vi "Uframe-Basler-MNR.vi"() -> ()   [LabVIEW 2010]
uses:
  <vilib>/userDefined/High Color/IMAQdx.ctl
  <vilib>/vision/driver/IMAQdx.llb/IMAQdx Buffer Number Mode.ctl
  <vilib>/Platform/TimedLoop/XDataNode/XDataNode.xnode
  <vilib>/Platform/TimedLoop/XDataNode/timing_clust.ctl
  <vilib>/Platform/TimedLoop/XDataNode/nitl_modes.ctl
  <vilib>/Platform/TimedLoop/XDataNode/wakeup.ctl
  <vilib>/Platform/TimedLoop/XDataNode/XDNodeRunTimeDep.lvlib
  <vilib>/vision/driver/NI_Vision_Acquisition_Software.lvlib
  Program Files/National Instruments/LabVIEW 2010/resource/objmgr/imaqdx.rc
panel:
  out "Load Cell Constant (N/V)":dbl=44.48
  in  "Load Cell":u16(ring)=1 items=["440 N", "1250 N"]
  in  "Pause @ Load":bool
  in  "Pause @ N":dbl
  out "Disp (mm)":dbl
  out "Load (N)":dbl
  out "Image #":i32
  in  "White Balance \nVR":dbl(slide)=1684.0 min=0.0 max=4095.0 step=1.0 scale=1.0..255.0 scale format="%#.0f"
  in  "White Balance\n UB":dbl(slide)=1684.0 min=0.0 max=4095.0 step=1.0 scale=1.0..255.0 scale format="%#.0f"
  in  "Illumination":u32(ring) items=["White Light", "Flourescent"]
  in  "Timed \nAcquisition":bool
  out "Data Point":i32
  in  "Shutter":dbl(slide)=20.0 min=0.0 max=4095.0 step=1.0 scale=4.095..4095.0 scale format="%#.0f"
  in  "Brightness":dbl(slide)=200.0 min=0.0 max=255.0 step=1.0 scale=0.0..255.0
  in  "Gain":dbl(slide)=702.0 min=350.0 max=1000.0 step=1.0 scale=350.0..1000.0
  in  "Video Mode Top":u32(ring)=47 items=["320x240 Color"=4, "640x480 Mono8"=9, "640x480 Mono16"=19, "640x480 Color"=14, "800x600 Mono8"=21, "800x600 Mono16"=27, "800x600 Color"=24, "1024x768 Mono8"=30, "1024x768 Mono16"=36, "1024x768 Color"=33, "1280x960 Mono8"=40, "1280x960 Mono16"=46, "1280x960 Color"=43, "1388x1038 Color"=47, "1388x1038 Mono"=48]
  in  "Session In Top View":T1="cam0"
  in  "Data \nAcquisition \nInterval (s)":dbl=1.0 min=0.1 max=60.0
  in  "Capture\nCurrent Image":bool
  out "Image":T2(plugin-control)
  in  "Max Load (N)":dbl=600.0 min=0.0 max=1200.0
  out "At Limit":bool
  in  "Rate Multiplier":dbl=1.0
  in  "Pause \nDisplacement":bool
  in  "Stop":bool
  in  "Invert \nDisplacement":bool
  in  "Zero \nDisplacement":bool=TRUE
  in  "Begin":bool
  out "Load vs Disp":cluster{dbl[], dbl[]}(graph)={[-724.1250113144533, -724.195323815552, -724.2656363166506, -724.3359488177492, -724.4062613188479, -724.4765738199465, -724.5468863210451, -724.6171988221438, -724.7461050741579, -724.9218863269045, -725.0976675796511, -725.2851675825808, -725.4492300851442], [-11.89350874713131, -11.896152101474941, -11.894229661847117, -11.89350874707076, -11.890865392620372, -11.895671491596438, -11.895911796524977, -11.899756675680168, -11.899035760801853, -11.90552399441818, -11.907927043887174, -11.905283689458143, -11.914655582386047]}
  out "Disp Vs Time":cluster{dbl[], dbl[]}(graph)={[-724.1250113144533, -724.195323815552, -724.2656363166506, -724.3359488177492, -724.4062613188479, -724.4765738199465, -724.5468863210451, -724.6171988221438, -724.7461050741579, -724.9218863269045, -725.0976675796511, -725.2851675825808, -725.4492300851442], [-11.89350874713131, -11.896152101474941, -11.894229661847117, -11.89350874707076, -11.890865392620372, -11.895671491596438, -11.895911796524977, -11.899756675680168, -11.899035760801853, -11.90552399441818, -11.907927043887174, -11.905283689458143, -11.914655582386047]}
  in  "File Name":string="Test"
  in  "File Path":path=path "C:/cygwin/home/Smarter Materials/Users 2015/Michael Rossol"
  in  "Sample Notes":string
  in  "Displacement \nRate (um/s)":dbl=3.0 min=3.0 max=50.0
  in  "Data Acquisition \nInterval (s)":dbl=1.0 min=0.1 max=10.0 step=0.01 format="%#_3g"
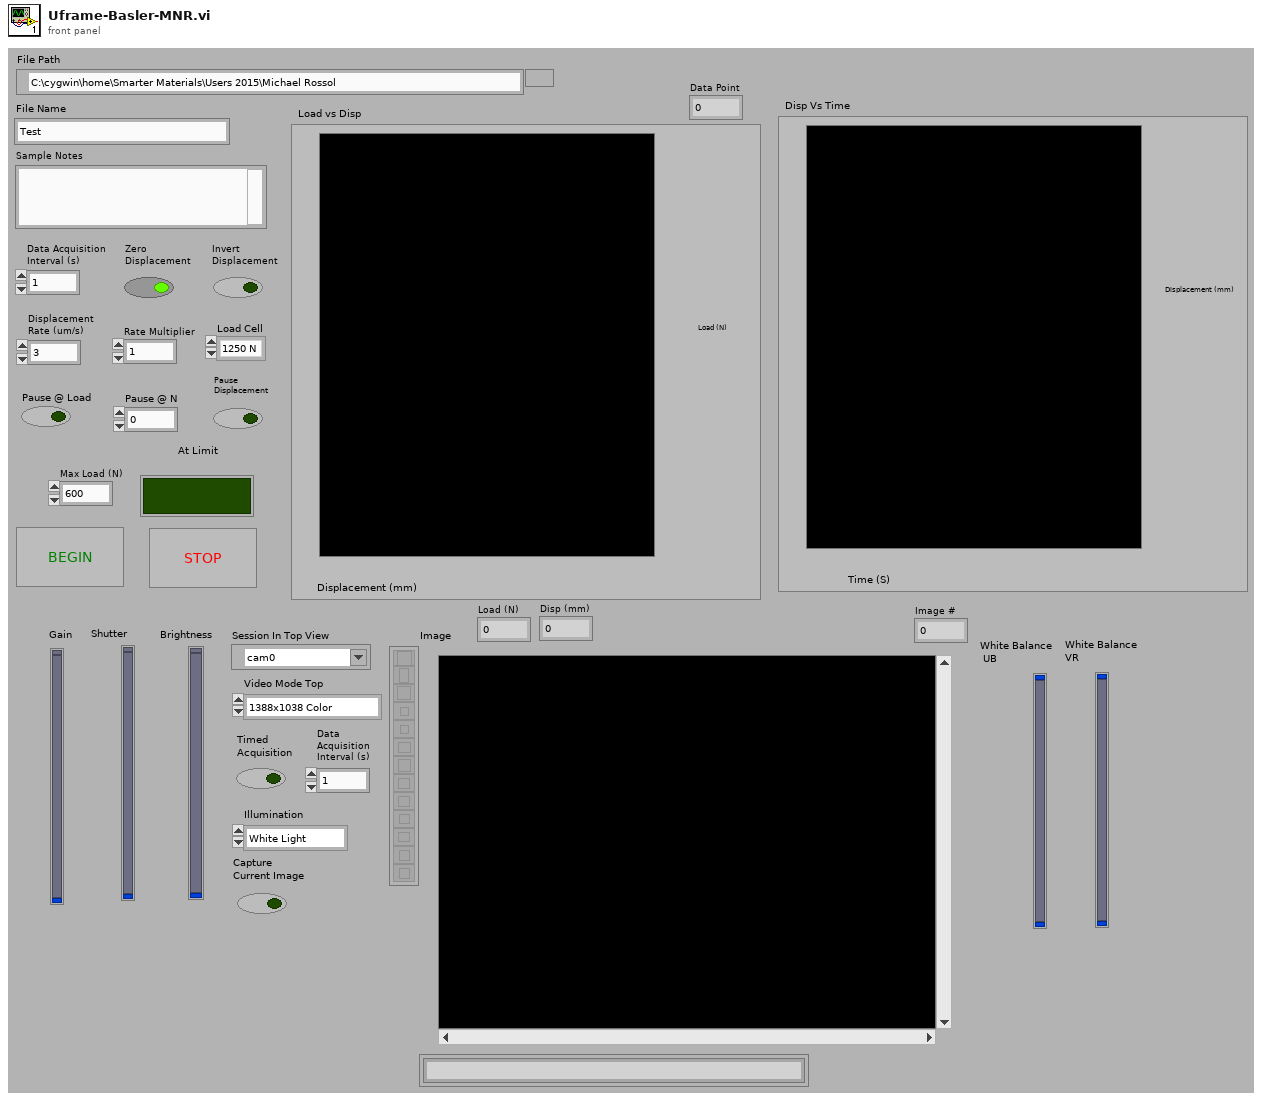
[diagram p1: front panel]
types:
  T1 = typedef "IMAQdx.ctl" = refnum<k21>
  T2 = typedef "IMAQ Image.ctl" = refnum<image>
  T3 = typedef "Image Type" = u32
  T4 = typedef "XDNodeRunTimeDep.lvlib/timing_clust.ctl" = cluster{"Expected End [f-1]":u64, "Actual End [f-1]":u64, "Finished Late? [f-1]":bool, "Expected End [i-1]":u64, "Actual End [i-1]":u64, "Finished Late? [i-1]":bool, "Expected Start [i]":u64, "Actual Start [i]":u64, "Expected Start [f]":u64, "Actual Start [f]":u64, "Source Name":string, "Structure Name":string, "Period":i64, "Deadline":i64, "Offset":i64, "Start":i64, "Priority":i32, "Timeout":i32, "Mode":T5, "Wakeup Reason":T6, "Error":errorcluster, "Source Type":string, "Secondary Source Type":string, "Global End Time":u64, "Global Start Time":u64, "Frame Duration":u64, "Iteration Duration":u64, "Assigned CPU":i32, "I/O Scan Engine Mode":u32}
  T5 = typedef "XDNodeRunTimeDep.lvlib/nitl_modes.ctl" = enum32{"No Change", "Process missed periods, maintain original phase", "Discard missed periods, maintain original phase", "Process missed periods, ignore original phase", "Discard missed periods, ignore original phase"}
  T6 = typedef "XDNodeRunTimeDep.lvlib/wakeup.ctl" = enum32{"Normal", "Aborted", "Asynchronous wakeup", "Timing source error", "Timed loop error", "Timeout"}
  T7 = typedef "NI_Vision_Acquisition_Software.lvlib/IMAQdx Buffer Number Mode.ctl" = enum32{"Next", "Last", "Buffer Number"}
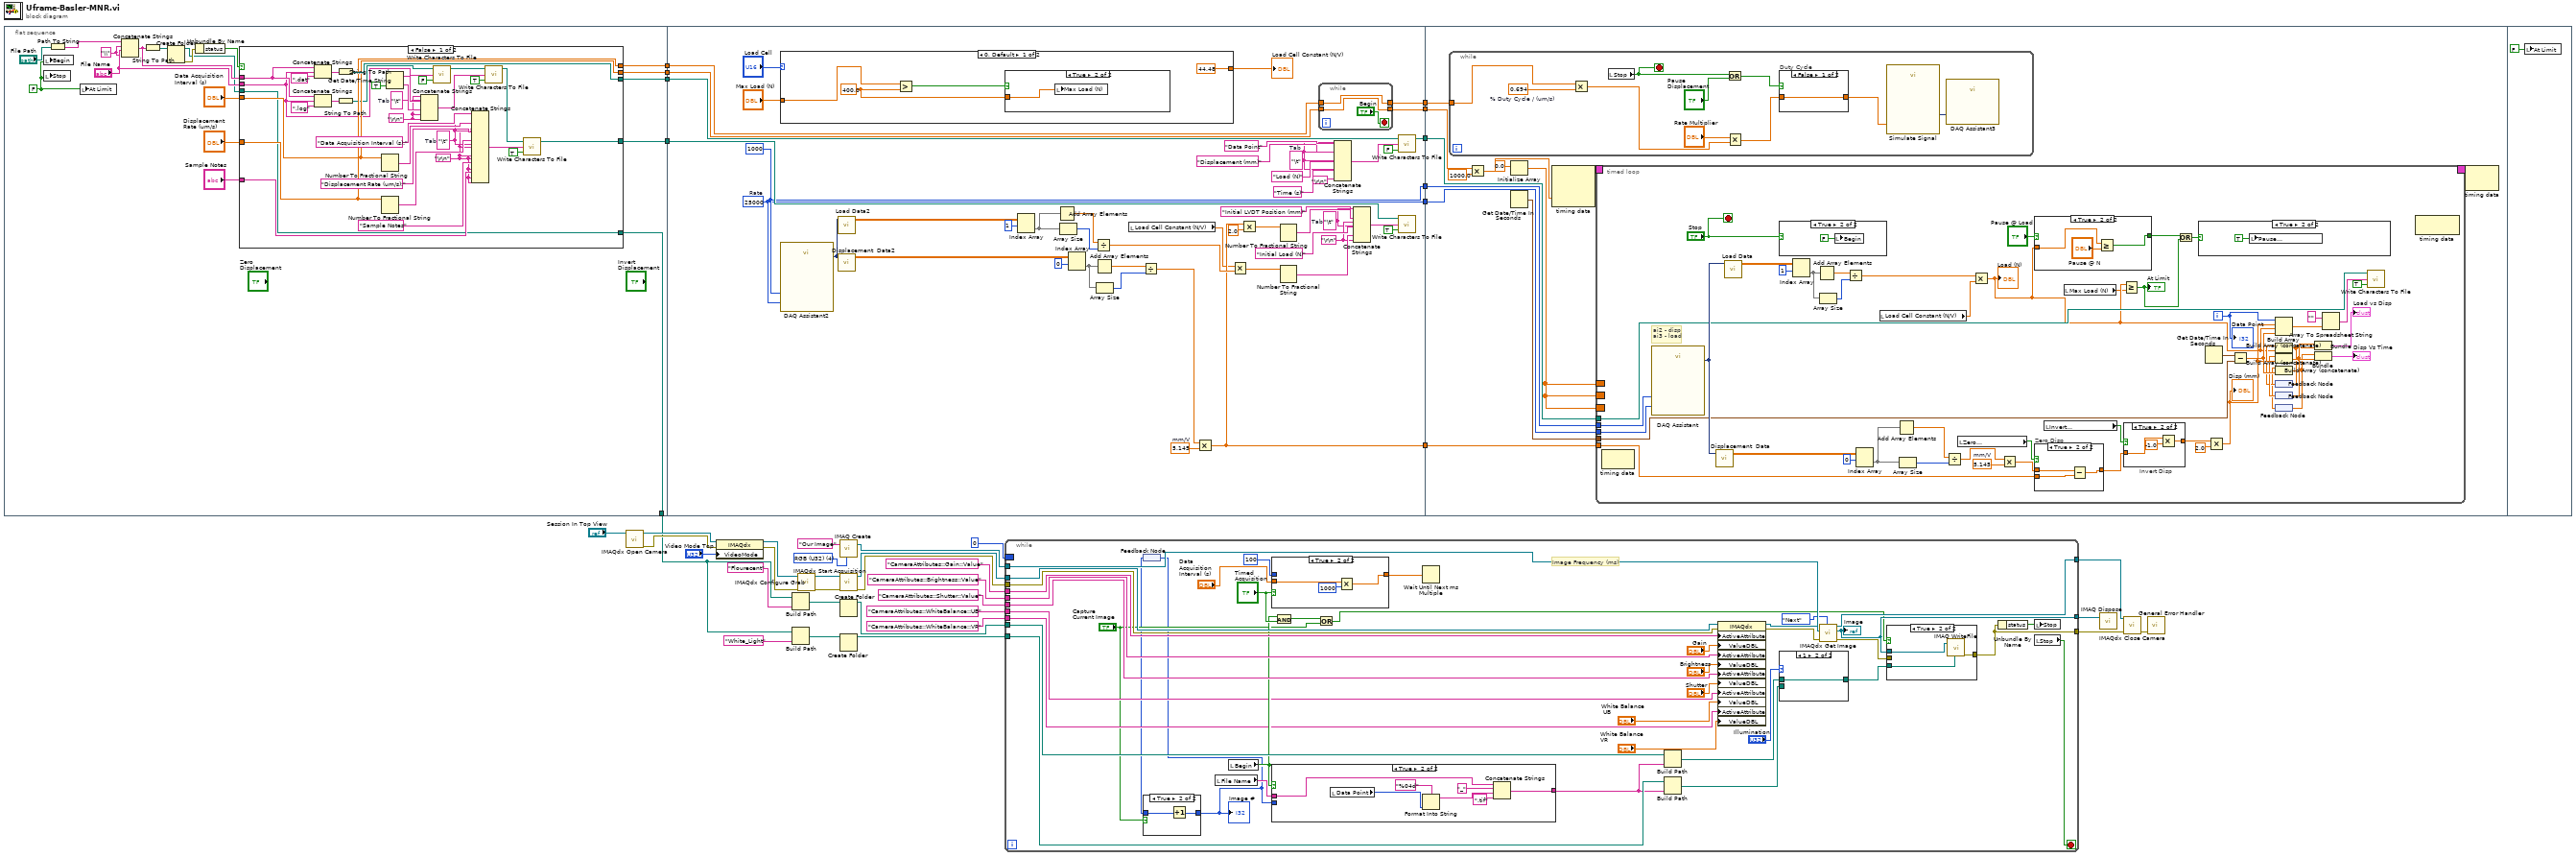
[diagram p0: block diagram]
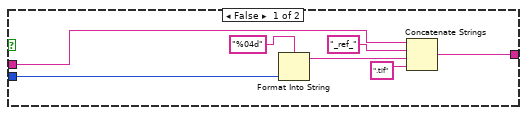
[diagram p3: hidden frame]
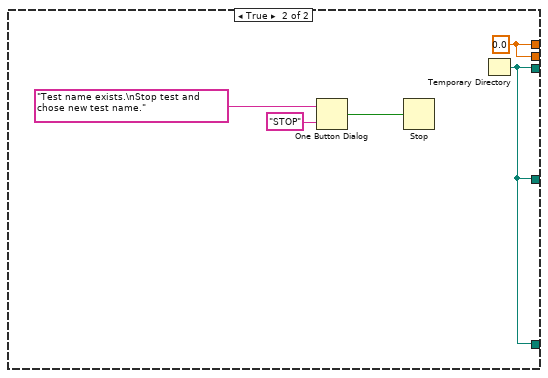
[diagram p7: hidden frame]
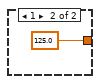
[diagram p9: hidden frame]
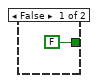
[diagram p10: hidden frame]
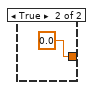
[diagram p15: hidden frame]
diagram:
  w26 = T3 4 items=["Grayscale (U8)", "Grayscale (I16)", "Grayscale (SGL)", "Complex (CSG)", "RGB (U32)", "HSL (U32)", "RGB (U64)"] ("Image Type")
  n1 = flat-sequence {
    tunnel: [w45] -> w36
    tunnel: [w57] -> w34
    tunnel: [w46] -> w33
    tunnel: [w47] -> w31
    tunnel: [w43] -> w5
    tunnel: [w100] -> w40
    tunnel: [w101] -> w39
    tunnel: [w102] -> w38
    tunnel: [w107] -> w37
    tunnel: w36 -> [w121]
    tunnel: [w112] -> w35
    tunnel: w34 -> [w111]
    tunnel: w33 -> [w104]
    tunnel: [w103] -> w32
    tunnel: w31 -> [w105]
    tunnel: w40 -> [w153]
    tunnel: w39 -> [w164]
    tunnel: w38 -> [w163]
    tunnel: w37 -> [w162]
    tunnel: w35 -> [w161]
    tunnel: w32 -> [w160]
    frame #0 {
      w44 = FALSE ("Begin")
      w42 = "\\"
      n2 = local write "Begin"(w44) -> ()
      n3 = local write "Stop"(w44) -> ()
      n4 = Path To String(path="File Path") -> (string=w52:string)
      n5 = local write "At Limit"(w44) -> ()
      n6 = Concatenate Strings(w52, w42, "File Name", w42) -> (w50:string)
      n7 = String To Path(string=w50) -> (path=w54:path)
      n8 = Create Folder(path (use dialog)=w54) -> (created path=w41:path, error out=w53:errorcluster)  [unwired: 2 in, 1 out]
      n9 = Unbundle By Name(w53) -> ("status"=w51:bool)
      n10 = case shown="False" w51 {
        tunnel: [w76 w92] -> w45
        tunnel: "Data Acquisition \nInterval (s)" -> [w71 _]
        tunnel: "Displacement \nRate (um/s)" -> [w72 _]
        tunnel: "Sample Notes" -> [w68 _]
        tunnel: [w73 w92] -> w57
        tunnel: [w72 w91] -> w46
        tunnel: [w71 w91] -> w47
        tunnel: w50 -> [w61 _]
        tunnel: "File Name" -> [w60 _]
        tunnel: [w59 w92] -> w43
        tunnel: w41 -> [w59 _]
        frame False {
          w70 = "\t"  # Tab
          w67 = "\r\n"
          w86 = "\t"  # Tab
          w81 = "\r\n"
          n11 = Concatenate Strings(w61, w60, ".dat") -> (w74:string)
          n12 = Concatenate Strings(w61, w60, ".log") -> (w63:string)
          n13 = String To Path(string=w74) -> (path=w73:path)
          n14 = String To Path(string=w63) -> (path=w62:path)
          n15 = Number To Fractional String(number=w71) -> (F-format string=w79:string)  [unwired: 3 in]
          n16 = Number To Fractional String(number=w72) -> (F-format string=w77:string)  [unwired: 3 in]
          n17 = Get Date/Time String(want seconds? (F)=TRUE) -> (date string=w89:string, time string=w88:string)  [unwired: 2 in]
          n18 = Concatenate Strings(w81, w89, w86, w88, w81, w81) -> (w90:string)
          n19 = call <vilib>:"Write Characters To File.vi"("append to file? (new file:F)"=FALSE, "character string"=w60, "file path (dialog if empty)"=w62) -> ("new file path (Not A Path if cancelled)"=w66:path)  [unwired: 2 in]
          n20 = Concatenate Strings("Data Acquisition Interval (s):", w70, w79, w67, "Displacement Rate (um/s):", w70, w77, w67, w70, w67, w67, "Sample Notes", w67, w68, w67, w67) -> (w82:string)
          n21 = call <vilib>:"Write Characters To File.vi"("append to file? (new file:F)"=TRUE, "character string"=w90, "file path (dialog if empty)"=w66) -> ("new file path (Not A Path if cancelled)"=w84:path)  [unwired: 2 in]
          n22 = call <vilib>:"Write Characters To File.vi"("append to file? (new file:F)"=TRUE, "character string"=w82, "file path (dialog if empty)"=w84) -> ("new file path (Not A Path if cancelled)"=w76:path)  [unwired: 2 in]
        }
        frame True {
          w91 = 0.0 ("Displacement Rate (um/s)")
          n23 = One Button Dialog(message="Test name exists.\nStop test and chose new test name.", button name ("OK")="STOP") -> (true=w93:bool)
          n24 = Stop(stop? (T)=w93) -> ()
          n25 = Temporary Directory() -> (w92:path)
        }
      }
    }
    frame #1 {
      w102 = 1000 ("number of samples")
      w114 = "\t"  # Tab
      w125 = "\r\n"
      w123 = "\t"  # Tab
      w139 = 5.145  # mm/V
      w101 = 25000  # Rate
      n26 = case shown="0, Default" "Load Cell" {
        tunnel: [44.48 125.0] -> w98
        tunnel: "Max Load (N)" -> [w144 _]
        frame 0, Default {
          w143 = 400.0 ("y")
          n27 = Greater?(x=w144, y=w143) -> (0:w145:bool)
          n28 = case shown="True" w145 {
            tunnel: w143 -> [_ w147]
            frame False {
            }
            frame True {
              n29 = local write "Max Load (N)"(w147) -> ()
            }
          }
        }
        frame 1 {
        }
      }
      "Load Cell Constant (N/V)" <- w98
      n30 = call "DAQ Assistant2"("rate"=w101, "number of samples"=w102) -> ("data"=w130:dynamicdata)  [unwired: 15 in, 2 out]
      n31 = call "Load Data2"("Dynamic Data Type"=w130) -> ("Array"=w131:dbl[][])  [unwired: 3 in]
      n32 = call "Displacement  Data2"("Dynamic Data Type"=w130) -> ("Array"=w134:dbl[][])  [unwired: 3 in]
      n33 = Index Array(array=w131, index (row)=1) -> (element=w142:dbl[])  [unwired: 1 in]
      n34 = Add Array Elements(numeric array=w142) -> (sum=w140:dbl)
      n35 = Array Size(array=w142) -> (size(s)=w141:i32)
      n36 = Index Array(array=w134, index (row)=0) -> (element=w135:dbl[])  [unwired: 1 in]
      n37 = Divide(x=w140, y=w141) -> (x/y=w109:dbl)
      n38 = Add Array Elements(numeric array=w135) -> (sum=w136:dbl)
      n39 = Array Size(array=w135) -> (size(s)=w137:i32)
      n40 = local read "Load Cell Constant (N/V)"() -> (w99:dbl)
      n41 = Divide(x=w136, y=w137) -> (x/y=w138:dbl)
      n42 = Multiply(x=w138, y=w139) -> (x*y=w107:dbl)
      n43 = Multiply(x=w99, y=w109) -> (x*y=w110:dbl)
      n44 = Multiply(x=w107, y=2.0) -> (x*y=w108:dbl)
      n45 = Number To Fractional String(number=w108) -> (F-format string=w124:string)  [unwired: 3 in]
      n46 = Number To Fractional String(number=w110) -> (F-format string=w127:string)  [unwired: 3 in]
      n47 = while {
        tunnel: w104 -> [w150]
        tunnel: [w150] -> w103
        tunnel: [w149] -> w100
        tunnel: w105 -> [w149]
        stop <- "Begin" stop-if-true
      }
      n48 = Concatenate Strings("Data Point", w114, "Displacement (mm)" ("Substring"), w114, "Load (N)", w114, "Time (s)" ("string"), w114, "\r\n") -> (w119:string)
      n49 = Concatenate Strings("Initial LVDT Position (mm)", w123, w124, w125, "Initial Load (N)", w123, w127, w125) -> (w128:string)
      n50 = call <vilib>:"Write Characters To File.vi"("append to file? (new file:F)"=FALSE, "character string"=w119, "file path (dialog if empty)"=w111) -> ("new file path (Not A Path if cancelled)"=w112:path)  [unwired: 2 in]
      n51 = call <vilib>:"Write Characters To File.vi"("append to file? (new file:F)"=TRUE, "character string"=w128, "file path (dialog if empty)"=w121) -> ()  [unwired: 2 in, 1 out]
    }
    frame #2 {
      n52 = while {
        tunnel: w160 -> [w241]
        stop <- w234 stop-if-true
        w235 = 0.694  # % Duty Cycle / (um/s)
        n53 = Multiply(x=w241, y=w235) -> (x*y=w238:dbl)
        n54 = local read "Stop"() -> (w234:bool)
        n55 = Or(x=w234, y="Pause \nDisplacement") -> (x .or. y?=w240:bool)
        n56 = Multiply(x="Rate Multiplier", y=w238) -> (x*y=w237:dbl)
        n57 = case "Duty Cycle" shown="False" w240 {
          tunnel: [w244 0.0 ("Duty Cycle (%)")] -> w242
          tunnel: w237 -> [w244 _]
          frame False {
          }
          frame True {
          }
        }
        n58 = call "Simulate Signal"("Duty Cycle (%)"=w242) -> ("Square"=w243:dynamicdata)  [unwired: 13 in, 1 out]
        n59 = call "DAQ Assistant3"("data"=w243) -> ()  [unwired: 16 in, 3 out]
      }
      n60 = Multiply(x=w153, y=1000.0) -> (x*y=w154:dbl)
      n61 = Get Date/Time In Seconds() -> (seconds since 1Jan1904=w157:timestamp)
      n62 = Initialize Array(0.0) -> (w158:dbl[])  [unwired: 1 in]
      n63 = node-c288(w154) -> (w156:T4)  [unwired: 2 in]
      n64 = timed-loop {
        tunnel: w163 -> [w196]
        tunnel: w164 -> [w195]
        tunnel: w162 -> [w187]
        tunnel: w157 -> [w191]
        tunnel: w161 -> [w190]
        border: w158 -> [_]
        border: w158 -> [_]
        border: w158 -> [_]
        timing: w156 -> [_]
        timing-out: [_] -> w155
        i -> [w173]
        stop <- "Stop" stop-if-true
        w194 = 5.145  # mm/V
        # "ai2 - disp\nai3 - load"
        n65 = node-c288() -> ()  [unwired: 1 in, 1 out]
        n66 = call "DAQ Assistant"("rate"=w195, "number of samples"=w196) -> ("data"=w193:dynamicdata)  [unwired: 15 in, 2 out]
        n67 = call "Displacement  Data"("Dynamic Data Type"=w193) -> ("Array"=w205:dbl[][])  [unwired: 3 in]
        n68 = call "Load Data"("Dynamic Data Type"=w193) -> ("Array"=w208:dbl[][])  [unwired: 3 in]
        n69 = case shown="True" "Stop" {
          frame False {
          }
          frame True {
            n70 = local write "Begin"(FALSE ("Begin")) -> ()
          }
        }
        n71 = Index Array(array=w208, index (row)=1) -> (element=w197:dbl[])  [unwired: 1 in]
        n72 = Add Array Elements(numeric array=w197) -> (sum=w199:dbl)
        n73 = Array Size(array=w197) -> (size(s)=w198:i32)
        n74 = Divide(x=w199, y=w198) -> (x/y=w184:dbl)
        n75 = Index Array(array=w205, index (row)=0) -> (element=w203:dbl[])  [unwired: 1 in]
        n76 = local read "Load Cell Constant (N/V)"() -> (w166:dbl)
        n77 = Add Array Elements(numeric array=w203) -> (sum=w202:dbl)
        n78 = Array Size(array=w203) -> (size(s)=w201:i32)
        n79 = Divide(x=w202, y=w201) -> (x/y=w200:dbl)
        n80 = local read "Zero \nDisplacement"() -> (w185:bool)
        n81 = Multiply(x=w184, y=w166) -> (x*y=w168:dbl)
        "Load (N)" <- w168
        n82 = Multiply(x=w200, y=w194) -> (x*y=w189:dbl)
        n83 = case shown="True" "Pause @ Load" {
          tunnel: w168 -> [_ w216]
          tunnel: [FALSE w215] -> w167
          frame False {
          }
          frame True {
            n84 = Greater Or Equal?(x=w216, y="Pause @ N") -> (x >= y?=w215:bool)
          }
        }
        n85 = case "Zero Disp" shown="True" w185 {
          tunnel: w187 -> [_ w229]
          tunnel: w189 -> [w226 w228]
          tunnel: [w226 w227] -> w188
          frame False {
          }
          frame True {
            n86 = Subtract(x=w228, y=w229) -> (x-y=w227:dbl)
          }
        }
        n87 = local read "Invert \nDisplacement"() -> (w186:bool)
        n88 = local read "Max Load (N)"() -> (w165:dbl)
        n89 = Greater Or Equal?(x=w168, y=w165) -> (x >= y?=w170:bool)
        "At Limit" <- w170
        n90 = case "Invert Disp" shown="True" w186 {
          tunnel: w188 -> [w222 w225]
          tunnel: [w222 w224] -> w182
          frame False {
          }
          frame True {
            n91 = Multiply(x=w225, y=-1.0) -> (x*y=w224:dbl)
          }
        }
        n92 = Or(x=w167, y=w170) -> (x .or. y?=w171:bool)
        n93 = case shown="True" w171 {
          frame False {
          }
          frame True {
            n94 = local write "Pause \nDisplacement"(TRUE ("Pause \nDisplacement")) -> ()
          }
        }
        n95 = Get Date/Time In Seconds() -> (seconds since 1Jan1904=w204:timestamp)
        n96 = Multiply(x=w182, y=2.0) -> (x*y=w181:dbl)
        "Disp (mm)" <- w181
        n97 = Subtract(x=w204, y=w191) -> (x-y=w192:dbl)
        n98 = Build Array(w173, w181, w168, w192) -> (w210:dbl[])
        n99 = feedback #1() -> (w176:dbl[])
        n100 = Build Array (concatenate)(w176, w168) -> (w177:dbl[])
        n101 = feedback-in #1(w177) -> ()
        n102 = feedback #2() -> (w178:dbl[])
        n103 = Build Array (concatenate)(w178, w181) -> (w179:dbl[])
        n104 = feedback-in #2(w179) -> ()
        n105 = feedback #3() -> (w174:dbl[])
        n106 = Build Array (concatenate)(w174, w192) -> (w175:dbl[])
        n107 = feedback-in #3(w175) -> ()
        n108 = Bundle(w179, w177) -> (→"Load vs Disp":cluster{dbl[], dbl[]})  [unwired: 1 in]
        n109 = Bundle(w175, w179) -> (→"Disp Vs Time":cluster{dbl[], dbl[]})  [unwired: 1 in]
        n110 = Array To Spreadsheet String(array=w210, 3:"" ("format string")) -> (spreadsheet string=w212:string)  [unwired: 1 in]
        n111 = call <vilib>:"Write Characters To File.vi"("append to file? (new file:F)"=TRUE, "character string"=w212, "file path (dialog if empty)"=w190) -> ()  [unwired: 2 in, 1 out]
        n112 = node-c288() -> ()  [unwired: 1 in, 1 out]
        "Data Point" <- w173
      }
      n113 = node-c288(w155) -> ()  [unwired: 1 out]
    }
    frame #3 {
      n114 = local write "At Limit"(FALSE ("Begin")) -> ()
    }
  }
  n115 = call <vilib>:"IMAQdx Open Camera.vi"("Session In"="Session In Top View") -> ("error out"=w24:errorcluster, "Session Out"=w25:T1)  [unwired: 9 in]
  n116 = property class="IMAQdx"(reference=w25, error in=w24, "VideoMode"="Video Mode Top") -> (reference out=w22:T1, error out=w23:errorcluster)
  n117 = Build Path(base path=w5, name or relative path="Flourecent") -> (appended path=w6:path)
  n118 = Build Path(base path=w5, name or relative path="White_Light") -> (appended path=w9:path)
  n119 = call <vilib>:"IMAQdx Configure Grab.vi"("error in"=w23, "Session In"=w22) -> ("error out"=w20:errorcluster, "Session Out"=w21:T1)  [unwired: 8 in]
  n120 = call "IMAQ Create"("Image Name"="Our Image", "Image Type"=w26) -> ("New Image"=w17:T2)  [unwired: 3 in, 1 out]
  n121 = call <vilib>:"IMAQdx Start Acquisition.vi"("error in"=w20, "Session In"=w21) -> ("error out"=w11:errorcluster, "Session Out"=w18:T1)  [unwired: 8 in]
  n122 = Create Folder(path (use dialog)=w6) -> (created path=w4:path)  [unwired: 2 in, 2 out]
  n123 = Create Folder(path (use dialog)=w9) -> (created path=w8:path)  [unwired: 2 in, 2 out]
  n124 = while {
    tunnel: w17 -> [w283]
    tunnel: "CameraAttributes::Gain::Value" ("ActiveAttribute") -> [w286]
    tunnel: "CameraAttributes::Brightness::Value" ("ActiveAttribute") -> [w285]
    tunnel: "CameraAttributes::Shutter::Value" ("ActiveAttribute") -> [w284]
    tunnel: [w277] -> w30
    tunnel: w11 -> [w281]
    tunnel: [w276] -> w29
    tunnel: w18 -> [w278]
    tunnel: [w274] -> w12
    tunnel: w8 -> [w268]
    tunnel: w4 -> [w266]
    tunnel: "CameraAttributes::WhiteBalance::UB" ("ActiveAttribute") -> [w253]
    tunnel: "CameraAttributes::WhiteBalance::VR" ("ActiveAttribute") -> [w252]
    border: 0 -> [_]
    stop <- w254 stop-if-true
    # "Image Frequency (ms)"
    n125 = feedback #4() -> (w248:i32)
    n126 = case shown="True" "Capture\nCurrent Image" {
      tunnel: w248 -> [w287 w289]
      tunnel: [w287 w288] -> w247
      frame False {
      }
      frame True {
        n127 = Increment(x=w289) -> (x+1=w288:i32)
      }
    }
    "Image #" <- w247
    n128 = feedback-in #4(w247) -> ()
    n129 = local read "File Name"() -> (w259:string)
    n130 = local read "Begin"() -> (w261:bool)
    n131 = case shown="True" "Timed \nAcquisition" {
      tunnel: u32 100 ("y") -> [w306 _]
      tunnel: [w306 w309] -> w272
      tunnel: "Data \nAcquisition \nInterval (s)" -> [_ w308]
      frame False {
      }
      frame True {
        n132 = Multiply(x=w308, y=1000) -> (x*y=w309:dbl)
      }
    }
    n133 = case shown="True" w261 {
      tunnel: [w294 w303] -> w260
      tunnel: w259 -> [w296 w302]
      tunnel: w247 -> [w292 _]
      frame False {
        n134 = Format Into String(format string="%04d", w292) -> (resulting string=w293:string)  [unwired: 2 in, 1 out]
        n135 = Concatenate Strings(w296, "_ref_" ("string"), w293, ".tif") -> (w294:string)
      }
      frame True {
        n136 = local read "Data Point"() -> (w297:i32)
        n137 = Format Into String(format string="%04d", w297) -> (resulting string=w299:string)  [unwired: 2 in, 1 out]
        n138 = Concatenate Strings(w302, "_" ("string"), w299, ".tif") -> (w303:string)
      }
    }
    n139 = And(x=w261, y="Timed \nAcquisition") -> (x .and. y?=w269:bool)
    n140 = Or(x=w269, y="Capture\nCurrent Image") -> (x .or. y?=w270:bool)
    n141 = Wait Until Next ms Multiple(millisecond multiple=w272) -> ()  [unwired: 1 out]
    n142 = Build Path(base path=w266, name or relative path=w260) -> (appended path=w263:path)
    n143 = Build Path(base path=w268, name or relative path=w260) -> (appended path=w265:path)
    n144 = property class="IMAQdx"(reference=w278, error in=w281, "ActiveAttribute"=w286, "ValueDBL"="Gain", "ActiveAttribute"=w285, "ValueDBL"="Brightness", "ActiveAttribute"=w284, "ValueDBL"="Shutter", "ActiveAttribute"=w253, "ValueDBL"="White Balance\n UB", "ActiveAttribute"=w252, "ValueDBL"="White Balance \nVR") -> (reference out=w280:T1, error out=w279:errorcluster)
    n145 = case shown="1" "Illumination" {
      tunnel: w265 -> [w304 _]
      tunnel: [w304 w305] -> w264
      tunnel: w263 -> [_ w305]
      frame 0, Default {
      }
      frame 1 {
      }
    }
    n146 = call <vilib>:"IMAQdx Get Image.vi"("Buffer Number Mode (Next)"=IMAQdx_Buffer_Number_Mode."Next", "error in"=w279, "Image In"=w283, "Session In"=w280) -> ("error out"=w275:errorcluster, "Image Out"=w274:T2, "Session Out"=w277:T1)  [unwired: 4 in, 1 out]
    "Image" <- w274
    n147 = case shown="True" w270 {
      tunnel: w274 -> [_ w313]
      tunnel: [w310 w312] -> w276
      tunnel: w264 -> [_ w311]
      tunnel: w275 -> [w310 _]
      frame False {
      }
      frame True {
        n148 = call "IMAQ WriteFile"("File Path"=w311, "Image"=w313) -> ("error out"=w312:errorcluster)  [unwired: 6 in]
      }
    }
    n149 = Unbundle By Name(w276) -> ("status"=w255:bool)
    n150 = local write "Stop"(w255) -> ()
    n151 = local read "Stop"() -> (w254:bool)
  }
  n152 = call "IMAQ Dispose"("Image"=w12) -> ()  [unwired: 5 in, 1 out]
  n153 = call <vilib>:"IMAQdx Close Camera.vi"("error in"=w29, "Session In"=w30) -> ("error out"=w28:errorcluster)  [unwired: 9 in]
  n154 = call <vilib>:"General Error Handler.vi"("error in (no error)"=w28) -> ()  [unwired: 10 in, 5 out]
